vi "Read Location.vi"(8 "error in (no error)":errorcluster, 11 "Array Location Mailman in":refnum<class "Array Location Mailman.lvclass">) -> (0 "error out":errorcluster, 2 "Location":i32[](array[numeric]), 3 "Array Location Mailman out":refnum<class "Array Location Mailman.lvclass">)   [LabVIEW 2019, in "Array Location Mailman.lvclass"]
uses:
  Array Location Mailman.lvclass
  Array Location Mailman.lvclass/Array Location Mailman.ctl
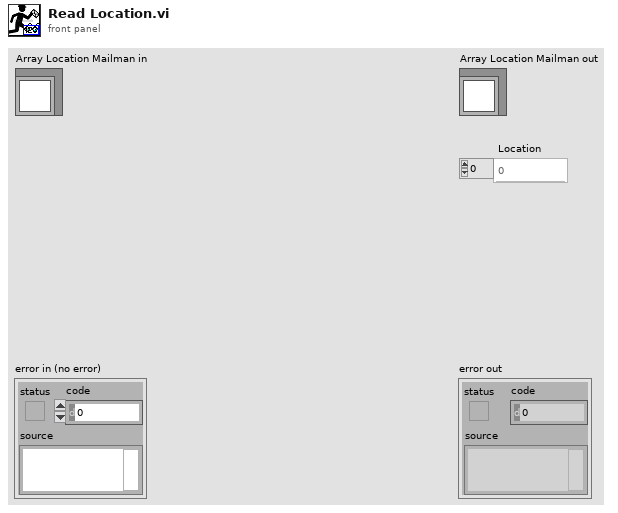
[diagram p1: front panel]
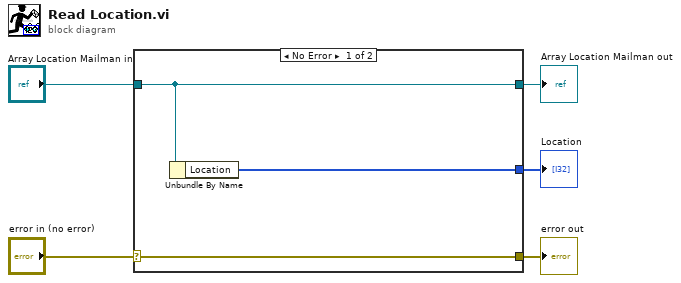
[diagram p0: block diagram]
diagram:
  n1 = case shown="No Error" "error in (no error)" {
    selector: "error in (no error)" -> [w8 w9]
    tunnel: [w8 w9] -> w4
    tunnel: [w7 w10] -> w2
    tunnel: "Array Location Mailman in" -> [w7 w10]
    tunnel: [w6 _] -> w1
    frame No Error {
      n2 = Unbundle By Name(w7) -> ("Location"=w6:i32[])
    }
    frame Error {
    }
  }
  "error out" <- w4
  "Array Location Mailman out" <- w2
  "Location" <- w1
